vi "Set Algorithm.vi"(8 "error in (no error)":errorcluster, 10 "Appliance":refnum<class "Appliance.lvclass">, 11 "Chef in":refnum<class "Chef.lvclass">) -> (0 "error out":errorcluster, 3 "Chef out":refnum<class "Chef.lvclass">)   [LabVIEW 2011, in "Chef.lvclass"]
uses:
  Chef.lvclass
  Appliance/Appliance.lvclass
  Chef.lvclass/Chef.ctl
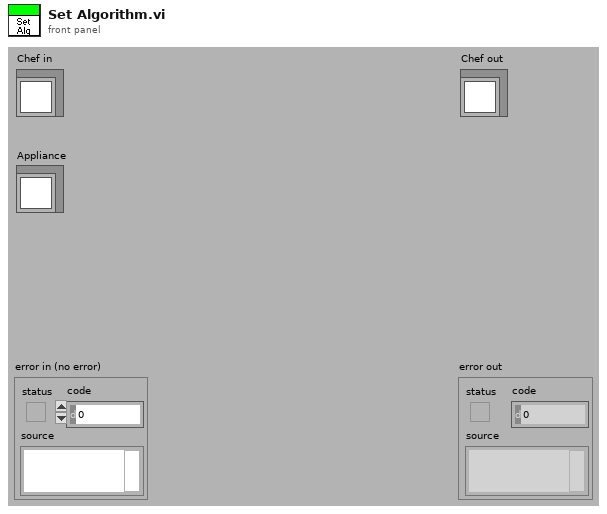
[diagram p1: front panel]
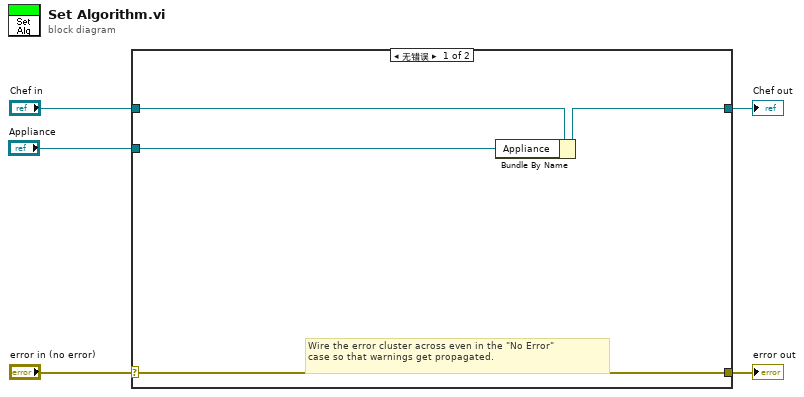
[diagram p0: block diagram]
diagram:
  n1 = case shown="无错误" "error in (no error)" {
    selector: "error in (no error)" -> [w8 w11]
    tunnel: [w8 w11] -> w4
    tunnel: [w7 w10] -> w2
    tunnel: "Chef in" -> [w9 w10]
    tunnel: "Appliance" -> [w6 _]
    frame No Error {
      # "Wire the error cluster across even in the \"No Error\"\ncase so that warnings get propagated."
      n2 = Bundle By Name(cluster=w9, "Appliance"=w6) -> (w7:refnum<class "Chef.lvclass">)
    }
    frame Error {
    }
  }
  "error out" <- w4
  "Chef out" <- w2
